vi "Example Threshold.vi"() -> ()   [LabVIEW 2013]
uses:
  C:/tf/play/labview/Tinkerforge.dll
  Tinkerforge.dll
panel:
  in  "stop":bool
  out "callback counter":i32
  out "last weight (g)":i32
  in  "uid":string="amb"
  in  "port":i32=4223
  in  "host":string="localhost"
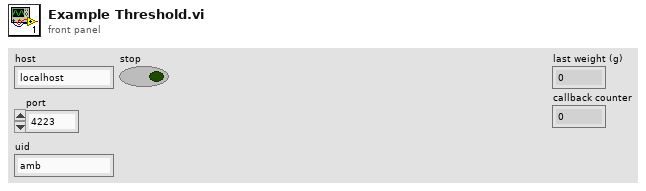
[diagram p1: front panel]
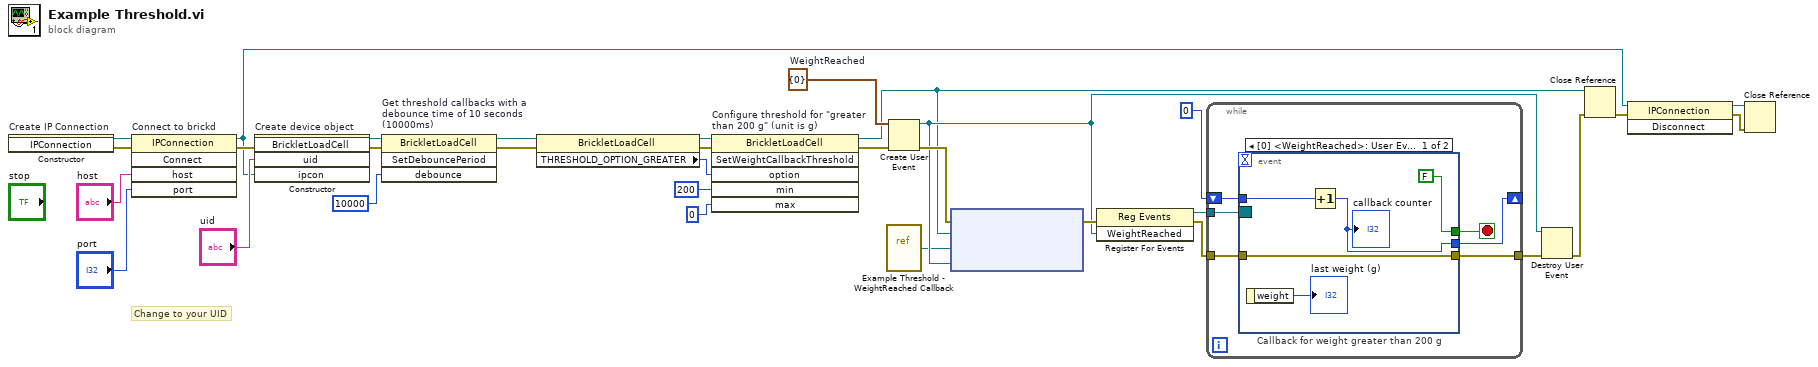
[diagram p0: block diagram]
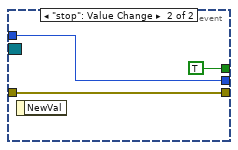
[diagram p2: hidden frame]
diagram:
  w16 = cluster{"weight":i32} {"weight"=0}  # WeightReached
  # "Change to your UID"
  n1 = constructor on="Create IP Connection" class="IPConnection"() -> (reference out=w32:refnum<k24>, error out=w1:errorcluster)  [unwired: 3 in, 1 out]
  n2 = invoke on="Connect to brickd" class="IPConnection" method="Connect"(reference=w32, error in=w1, "host"="host", "port"="port") -> (reference out=w25:refnum<k24>, error out=w28:errorcluster)  [unwired: 1 in, 3 out]
  n3 = constructor on="Create device object" class="BrickletLoadCell"(error in=w28, "uid"="uid", "ipcon"=w25) -> (reference out=w14:refnum<k24>, error out=w15:errorcluster)  [unwired: 2 in, 3 out]
  n4 = invoke on="Get threshold callbacks with a\ndebounce time of 10 seconds\n(10000ms)" class="BrickletLoadCell" method="SetDebouncePeriod"(reference=w14, error in=w15, "debounce"=i64 10000 ("period")) -> (reference out=w6:refnum<k24>, error out=w8:errorcluster)  [unwired: 1 in, 2 out]
  n5 = property class="BrickletLoadCell"(reference=w6, error in=w8) -> (reference out=w5:refnum<k24>, error out=w7:errorcluster, "THRESHOLD_OPTION_GREATER"=w4:u16)
  n6 = invoke on="Configure threshold for \"greater\nthan 200 g\" (unit is g)" class="BrickletLoadCell" method="SetWeightCallbackThreshold"(reference=w5, error in=w7, "option"=w4, "min"=200, "max"=0) -> (reference out=w12:refnum<k24>, error out=w11:errorcluster)  [unwired: 1 in, 4 out]
  n7 = vi-ref "Example Threshold - WeightReached Callback.vi"() -> ("vi reference"=w2:refnum<vi>)
  n8 = Create User Event(user event datatype=w16, error in=w11) -> (user event=w18:refnum<user-event>, error out=w23:errorcluster)
  n9 = node ("Register Event Callback")(w23, w12, w2, w18) -> (w22:errorcluster)  [unwired: 1 in, 1 out]
  n10 = register-events(error in=w22, w18) -> (reference out=w21:refnum<event-registration>, error out=w19:errorcluster)  [unwired: 1 in]
  n11 = while {
    tunnel: w21 -> [w38]
    tunnel: [w37] -> w20
    tunnel: w19 -> [w36]
    shift-right: [w34] -> _
    shift-left: 0 -> [w35]
    stop <- w33 stop-if-true
    n12 = event "Callback for weight greater than 200 g" shown="[0] <WeightReached>: User Event" {
      selector: w38 -> [_ _]
      dyn-events: _ -> [_ _]
      timeout: _ -> [_ _]
      tunnel: [w43 w45] -> w37
      tunnel: w36 -> [w43 w45]
      tunnel: w35 -> [w42 w44]
      tunnel: [w41 w44] -> w34
      tunnel: [FALSE TRUE] -> w33
      event User Event {
        n13 = event-data() -> ("weight"=→"last weight (g)":i32)  [unwired: 1 in]
        n14 = Increment(x=w42) -> (x+1=w41:i32)
        "callback counter" <- w41
      }
      event "stop": Value Change {
        n15 = event-data() -> ()  [unwired: 1 in, 1 out]
      }
    }
  }
  n16 = Destroy User Event(user event=w18, error in=w20) -> (error out=w17:errorcluster)
  n17 = Close Reference(reference=w12, error in (no error)=w17) -> (error out=w27:errorcluster)
  n18 = invoke class="IPConnection" method="Disconnect"(reference=w25, error in=w27) -> (reference out=w24:refnum<k24>, error out=w26:errorcluster)  [unwired: 1 in, 1 out]
  n19 = Close Reference(reference=w24, error in (no error)=w26) -> ()  [unwired: 1 out]
